vi "数据查询_数据查询.vi"() -> ()   [LabVIEW 2016]
uses:
  <vilib>/Utility/miscctls.llb/LVPointTypeDef.ctl
  <vilib>/Utility/miscctls.llb/LVRowAndColumnUnsignedTypeDef.ctl
  <vilib>/addons/database/_DB Variant To Data/Database Variant To Data.xnode
panel:
  in  "工作模式":string(combo)="全部数据"
  out "连接的字符串":string
  out "选中数据表":string
  in  "查询":bool
  in  "结束日期":string="2020/01/01"
  in  "起始日期":string="2010/01/01"
  out "XY图":cluster{"data":timestamp[], "data":dbl[]}[](graph)
  in  "组合框":string(combo)
  out "数据表":string[][](table)
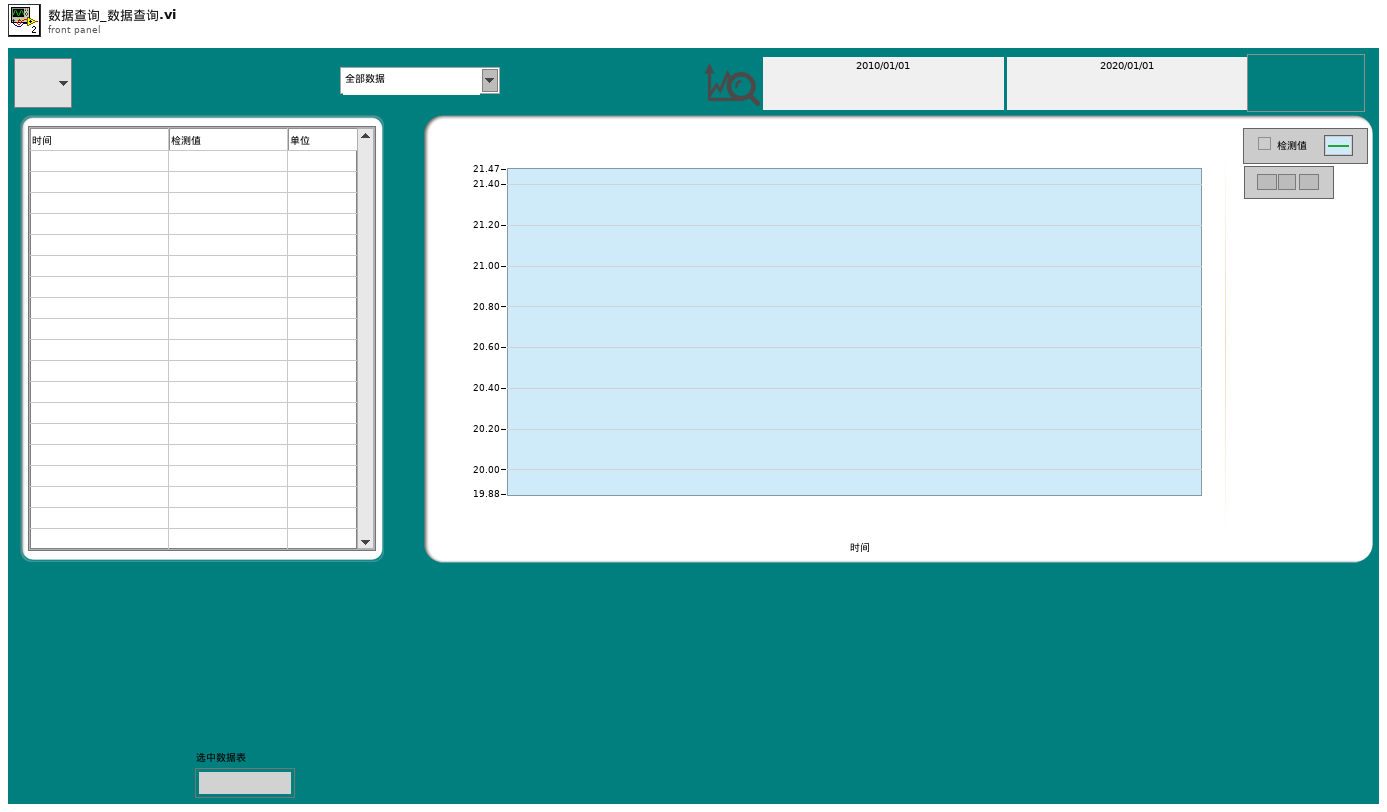
[diagram p1: front panel]
types:
  T1 = typedef "LVPointTypeDef.ctl" = cluster{"Horizontal":i16, "Vertical":i16}
  T2 = typedef "LVRowAndColumnUnsignedTypeDef.ctl" = cluster{"Row":u32, "Column":u32}
  T3 = typedef "LVPoint32TypeDef.ctl" = cluster{"Horizontal":i32, "Vertical":i32}
  T4 = typedef "LVPointDoubleTypeDef.ctl" = cluster{"Cursor X":dbl, "Cursor Y":dbl}
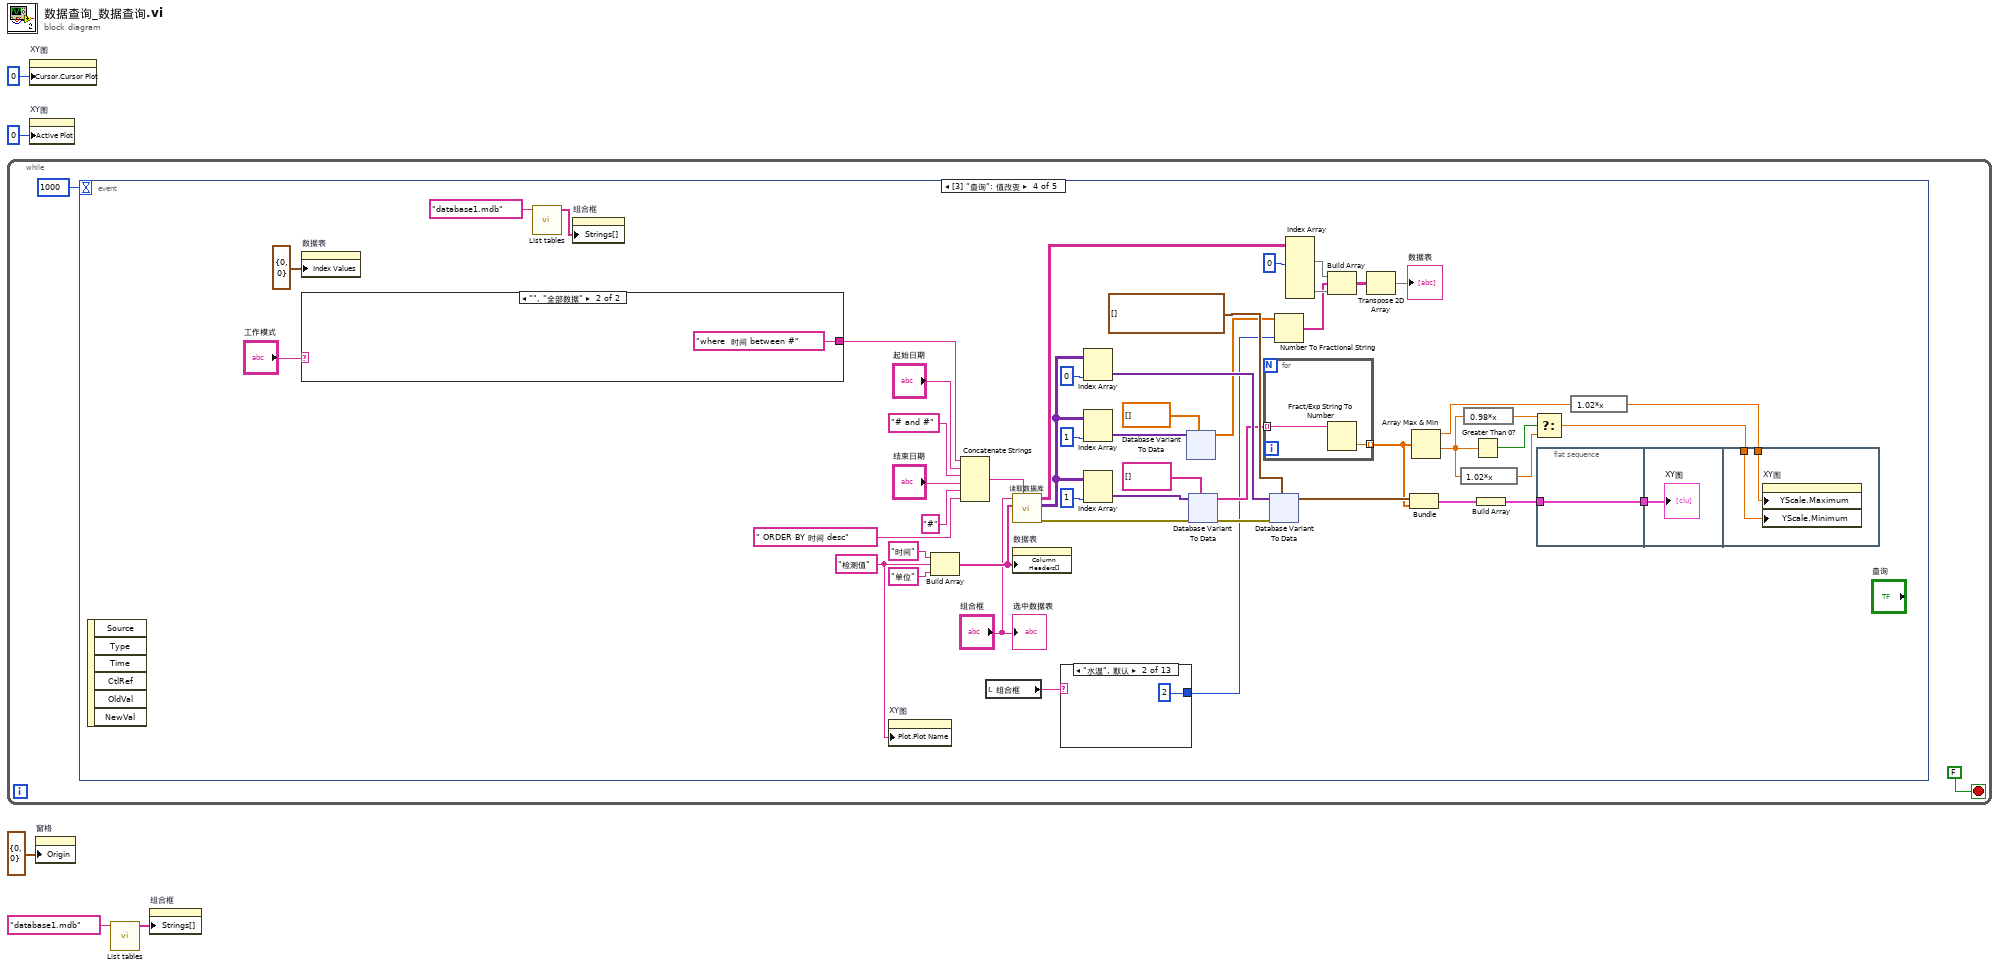
[diagram p0: block diagram]
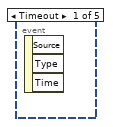
[diagram p2: hidden frame]
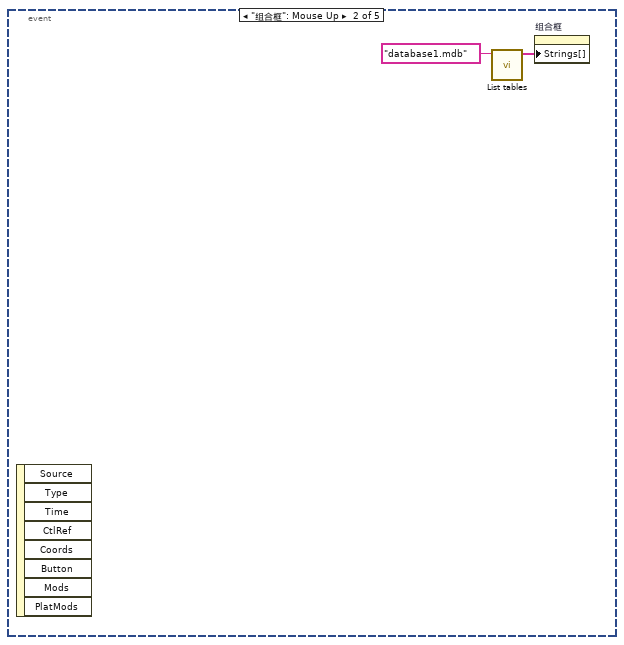
[diagram p3: hidden frame]
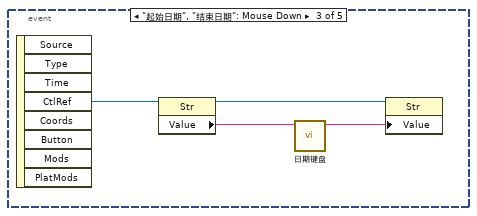
[diagram p4: hidden frame]
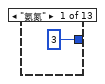
[diagram p5: hidden frame]
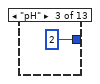
[diagram p6: hidden frame]
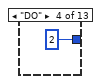
[diagram p7: hidden frame]
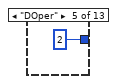
[diagram p8: hidden frame]
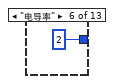
[diagram p9: hidden frame]
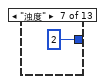
[diagram p10: hidden frame]
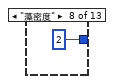
[diagram p11: hidden frame]
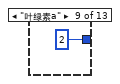
[diagram p12: hidden frame]
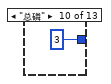
[diagram p13: hidden frame]
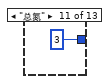
[diagram p14: hidden frame]
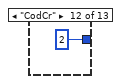
[diagram p15: hidden frame]
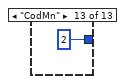
[diagram p16: hidden frame]
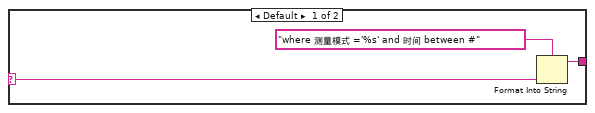
[diagram p17: hidden frame]
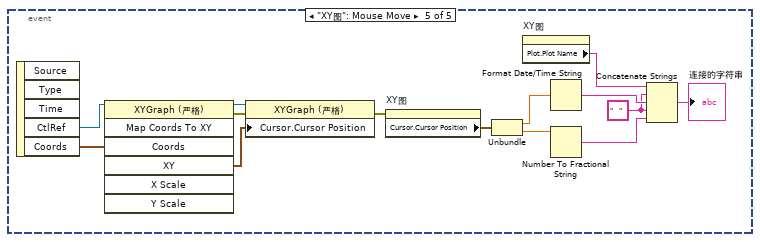
[diagram p18: hidden frame]
diagram:
  n1 = while {
    stop <- FALSE stop-if-true
    n2 = event shown="[3] \"查询\": 值改变" {
      selector: _ -> [_ _ _ _ _]
      dyn-events: _ -> [_ _ _ _ _]
      timeout: 1000 -> [_ _ _ _ _]
      event Timeout {
        n3 = event-data() -> ()  [unwired: 1 in, 3 out]
      }
      event "组合框": Mouse Up {
        n4 = event-data() -> ()  [unwired: 1 in, 8 out]
        n5 = call "List tables.vi"("database"="database1.mdb") -> ("tables"=w9:string[])  [unwired: 9 in, 1 out]
        n6 = property on="组合框" class="CmbBox"("Strings[]"=w9) -> ()  [unwired: 2 in, 2 out]
      }
      event "起始日期", "结束日期": Mouse Down {
        n7 = event-data() -> ("CtlRef"=w13:refnum<vi>)  [unwired: 1 in, 7 out]
        n8 = property class="Str"(reference=w13) -> (reference out=w11:refnum<vi>, "Value"=w12:string)  [unwired: 1 in, 1 out]
        n9 = call "日期键盘.vi"("原值"=w12) -> ("x+y"=w10:string)  [unwired: 10 in]
        n10 = property class="Str"(reference=w11, "Value"=w10) -> ()  [unwired: 1 in, 2 out]
      }
      event "查询": Value Change {
        w38 = "检测值"
        n11 = event-data() -> ()  [unwired: 1 in, 6 out]
        n12 = property on="数据表" class="Tbl (严格)"("Index Values"=T2 {"Row"=0, "Column"=0} ("索引值")) -> ()  [unwired: 2 in, 2 out]
        n13 = case shown="\"\", \"全部数据\"" "工作模式" {
          selector: "工作模式" -> [w80 _]
          tunnel: [w78 "where  时间 between #" ("condition")] -> w27
          frame Default {
            n14 = Format Into String(format string="where 测量模式 ='%s' and 时间 between #" ("condition"), w80) -> (resulting string=w78:string)  [unwired: 2 in, 1 out]
          }
          frame "", "全部数据" {
          }
        }
        n15 = call "List tables.vi"("database"="database1.mdb") -> ("tables"=w23:string[])  [unwired: 9 in, 1 out]
        n16 = property on="组合框" class="CmbBox"("Strings[]"=w23) -> ()  [unwired: 2 in, 2 out]
        n17 = property on="XY图" class="XYGraph (严格)"("Plot.Plot Name"=w38) -> ()  [unwired: 2 in, 2 out]
        n18 = Build Array("时间", w38, "单位" ("元素")) -> (w40:string[])
        n19 = Concatenate Strings(w27, "起始日期", "# and #" ("condition"), "结束日期", "#" ("condition"), " ORDER BY 时间 desc" ("字符串")) -> (w63:string)
        n20 = local read "组合框"() -> (w26:string)
        n21 = call "读取数据库.vi"("condition"=w63, "显示项"=w40, "组合框"="组合框") -> ("error out"=w54:errorcluster, "data"=w35:variant[][], "表格"=w46:string[][])  [unwired: 5 in, 1 out]
        n22 = property on="数据表" class="Tbl (严格)"("Column Headers[]"=w40) -> ()  [unwired: 2 in, 2 out]
        n23 = case shown="\"水温\", 默认" w26 {
          tunnel: [i16 3 ("精度(6)") i16 2 ("精度(6)") i16 2 ("精度(6)") i16 2 ("精度(6)") i16 2 ("精度(6)") i16 2 ("精度(6)") i16 2 ("精度(6)") i16 2 ("精度(6)") i16 2 ("精度(6)") i16 3 ("精度(6)") i16 3 ("精度(6)") i16 2 ("精度(6)") i16 2 ("精度(6)")] -> w25
          frame "氨氮" {
          }
          frame "水温", Default {
          }
          frame "pH" {
          }
          frame "DO" {
          }
          frame "DOper" {
          }
          frame "电导率" {
          }
          frame "浊度" {
          }
          frame "藻密度" {
          }
          frame "叶绿素a" {
          }
          frame "总磷" {
          }
          frame "总氮" {
          }
          frame "CodCr" {
          }
          frame "CodMn" {
          }
        }
        n24 = Index Array(array=w35, index (col)=0 ("禁用的索引 (列)")) -> (element=w57:variant[])  [unwired: 1 in]
        n25 = Index Array(array=w35, index (col)=1 ("禁用的索引 (列)")) -> (element=w33:variant[])  [unwired: 1 in]
        n26 = Index Array(array=w35, index (col)=1 ("禁用的索引 (列)")) -> (element=w55:variant[])  [unwired: 1 in]
        n27 = xnode "Database Variant To Data"("database variant"=w33, "type"=sgl[] []) -> ("data"=w31:sgl[])  [unwired: 1 in, 1 out]
        n28 = xnode "Database Variant To Data"("database variant"=w55, "error in (no error)"=w54, "type"=string[] []) -> ("data"=w39:string[], "error out"=w53:errorcluster)
        n29 = for {
          tunnel: w39 -> [w121] mode=indexing
          tunnel: [w120] -> w21 mode=indexing
          n30 = Fract/Exp String To Number(string=w121) -> (number=w120:dbl)  [unwired: 3 in, 1 out]
        }
        n31 = xnode "Database Variant To Data"("database variant"=w57, "error in (no error)"=w53, "type"=timestamp[] []) -> ("data"=w48:timestamp[])  [unwired: 1 out]
        n32 = Number To Fractional String(number=w31, precision (6)=w25) -> (F-format string=w30:string[])  [unwired: 2 in]
        n33 = Index Array(array=w46, index (col) #1=0 ("禁用的索引 (列)")) -> (element #1=w44:string[], element #3=w36:string[])  [unwired: 5 in, 1 out]
        n34 = Build Array(w44, w30, w36) -> (w43:string[][])
        n35 = Transpose 2D Array(2D array=w43) -> (transposed array=→"数据表":string[][])
        n36 = Bundle("data"=w48, w21) -> (w49:cluster{"data":timestamp[], dbl[]})  [unwired: 1 in]
        n37 = Array Max & Min(array=w21) -> (max value=w20:dbl, min value=w15:dbl)  [unwired: 2 out]
        n38 = expression code="1.02*x"(w15) -> (w16:dbl)
        n39 = expression code="0.98*x"(w15) -> (w17:dbl)
        n40 = Greater Than 0?(x=w15) -> (x > 0?=w18:bool)
        n41 = Build Array(w49) -> (w50:cluster{"data":timestamp[], dbl[]}[])
        n42 = Select(t=w17, s=w18, f=w16) -> (s? t:f=w14:dbl)
        n43 = flat-sequence {
          tunnel: [w122] -> w51
          tunnel: w50 -> [w122]
          tunnel: w51 -> [w123]
          tunnel: w14 -> [w125]
          tunnel: w19 -> [w124]
          frame #0 {
          }
          frame #1 {
            "XY图" <- w123
          }
          frame #2 {
            n44 = property on="XY图" class="XYGraph (严格)"("YScale.Maximum"=w124, "YScale.Minimum"=w125) -> ()  [unwired: 2 in, 2 out]
          }
        }
        n45 = expression code="1.02*x"(w20) -> (w19:dbl)
        "选中数据表" <- "组合框"
      }
      event "XY图": Mouse Move {
        w219 = "   " ("字符串")
        n46 = event-data() -> ("CtlRef"=w229:refnum<vi>, "Coords"=w228:T3)  [unwired: 1 in, 3 out]
        n47 = invoke class="XYGraph (严格)" method="Map Coords To XY"(reference=w229, "Coords"=w228) -> (reference out=w227:refnum<vi>, error out=w224:errorcluster, "XY"=w226:cluster{"X":dbl, "Y":dbl})  [unwired: 5 in, 4 out]
        n48 = property class="XYGraph (严格)"(reference=w227, error in=w224, "Cursor.Cursor Position"=w226) -> (error out=w225:errorcluster)  [unwired: 1 out]
        n49 = property on="XY图" class="XYGraph (严格)"(error in=w225) -> ("Cursor.Cursor Position"=w222:T4)  [unwired: 1 in, 2 out]
        n50 = Unbundle(w222) -> ("Cursor X"=w221:dbl, "Cursor Y"=w218:dbl)
        n51 = property on="XY图" class="XYGraph (严格)"() -> ("Plot.Plot Name"=w216:string)  [unwired: 2 in, 2 out]
        n52 = Format Date/Time String(seconds (now)=w221) -> (date/time string=w220:string)  [unwired: 2 in]
        n53 = Number To Fractional String(number=w218) -> (F-format string=w217:string)  [unwired: 3 in]
        n54 = Concatenate Strings(w216, w219, w220, w219, w217) -> (→"连接的字符串":string)
      }
    }
  }
  n55 = property on="XY图" class="XYGraph (严格)"("Cursor.Cursor Plot"=0 ("游标.游标关联曲线")) -> ()  [unwired: 2 in, 2 out]
  n56 = property on="XY图" class="XYGraph (严格)"("Active Plot"=u32 0 ("活动曲线")) -> ()  [unwired: 2 in, 2 out]
  n57 = property on="窗格" class="Pane"("Origin"=T1 {"Horizontal"=0, "Vertical"=0} ("原点")) -> ()  [unwired: 2 in, 2 out]
  n58 = call "List tables.vi"("database"="database1.mdb") -> ("tables"=w1:string[])  [unwired: 9 in, 1 out]
  n59 = property on="组合框" class="CmbBox"("Strings[]"=w1) -> ()  [unwired: 2 in, 2 out]
